vi "Subtract 1D and 2D Array.vi"(9 "2D Array":dbl[][](array[numeric]), 11 "1D Array":dbl[](array[numeric])) -> (2 "Diff Array":dbl[][](array[numeric]))   [LabVIEW 2020]
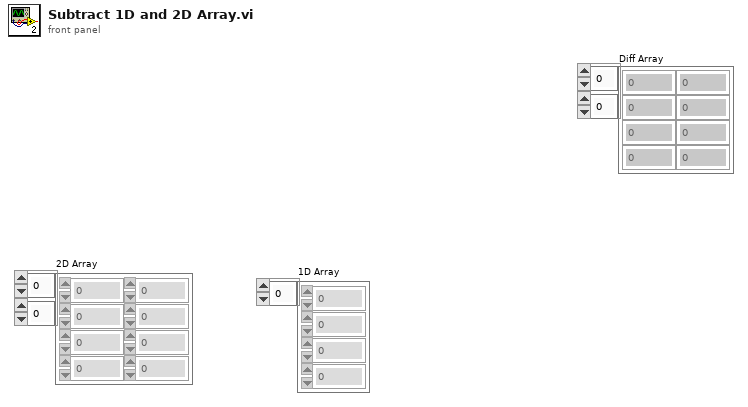
[diagram p1: front panel]
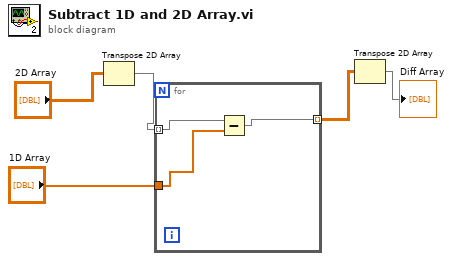
[diagram p0: block diagram]
diagram:
  n1 = Transpose 2D Array(2D array="2D Array") -> (transposed array=w3:dbl[][])
  n2 = for {
    tunnel: "1D Array" -> [w7]
    tunnel: w3 -> [w8] mode=indexing
    tunnel: [w6] -> w2 mode=indexing
    n3 = Subtract(x=w8, y=w7) -> (x-y=w6:dbl[])
  }
  n4 = Transpose 2D Array(2D array=w2) -> (transposed array=→"Diff Array":dbl[][])
